vi "ReversedEngineering GetControlInfo.vi"(2 "CtlRefnum":refnum<vi>, 3 "Default Value":variant, 5 "error in":errorcluster) -> (15 "attributeInfoType":T2={"name"="", "type"=enum."UINT8", "dimension"=0, "typeName"="", "typePath"=path "", "visibility"=enum."Protected"}, 19 "error out":errorcluster)   [LabVIEW 2020]
uses:
  <resource>/Framework/Providers/Open_GDS/UML/ReversedEngineering/ReversedEngineering AttributeInfoType.ctl
  <resource>/Framework/Providers/Open_GDS/ClassProviders/Common/CommonVIs/CommonVIs_AttributeDataType.ctl
  <resource>/Framework/Providers/Open_GDS/UML/UMLEditor/UMLEditor_VisibilityType.ctl
  <vilib>/numeric/LVNumericRepresentation.ctl
  <vilib>/Utility/Data Type/Type Definitions/Data Type.ctl
  <vilib>/Utility/Data Type/NI_Data Type.lvlib
panel:
  out "representation":T1
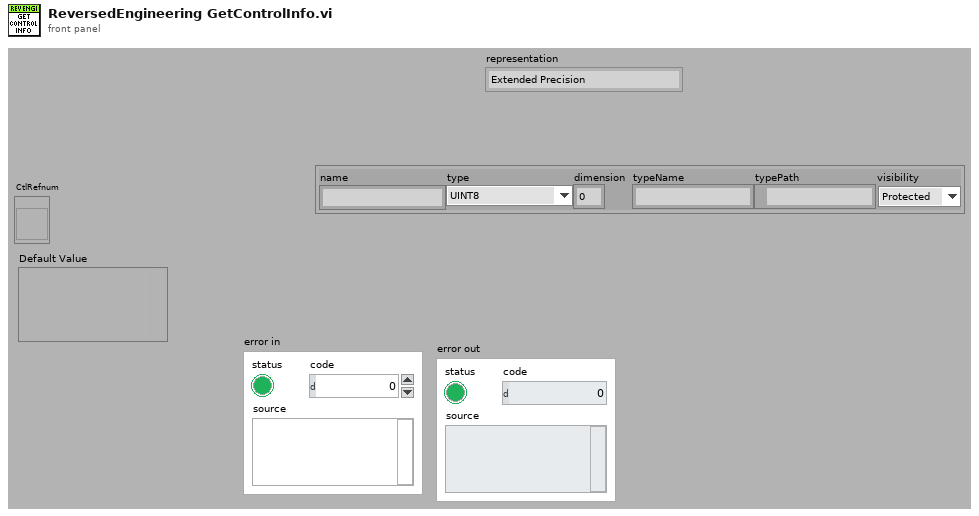
[diagram p1: front panel]
types:
  T1 = typedef "LVNumericRepresentation.ctl" = enum32{"Extended Precision", "Double Precision", "Single Precision", "Long", "Word", "Byte", "Unsigned Long", "Unsigned Word", "Unsigned Byte", "Complex Extended", "Complex Double", "Complex Single", "Quad", "Unsigned Quad", "Fixed-Point"}
  T2 = typedef "ReversedEngineering AttributeInfoType.ctl" = cluster{"name":string, "type":T3, "dimension":i32, "typeName":string, "typePath":path, "visibility":T4}
  T3 = typedef "CommonVIs_AttributeDataType.ctl" = enum16{"UINT8", "INT8", "UINT16", "INT16", "UINT32", "INT32", "UINT64", "INT64", "SGL", "DBL", "EXT", "CSG", "CDB", "CXT", "TimeStamp", "STRING", "PATH", "BOOL", "ENUM", "RefNum", "VIRefNum", "LabVIEW Class", "Cluster", "Variant", "TypeDef", "Waveform", "LabVIEW Object", "Other", "void", "Set", "Map"}
  T4 = typedef "UMLEditor_VisibilityType.ctl" = enum16{"Public", "Private", "Protected"}
  T5 = typedef "NI_Data Type.lvlib/Data Type.ctl" = enum8{"Invalid Type", "Void", "I8", "I16", "I32", "I64", "U8", "U16", "U32", "U64", "Single Float", "Double Float", "Extended Float", "Single Complex", "Double Complex", "Extended Complex", "Enum U8", "Enum U16", "Enum U32", "Enum U64", "Single Float With Unit", "Double Float With Unit", "Extended Float With Unit", "Single Complex with Unit", "Double Complex with Unit", "Extended Complex with Unit", "Boolean", "String", "Path", "Picture", "Tag", "Array", "Cluster", "Variant", "LV Variant", "Waveform", "Timestamp", "Digital Waveform", "Digital Data", "ExpressData", "Refnum", "External Data", "VI", "Poly VI", "LabVIEW Class Instance", "Fixed Point", "Set Collection", "Map Collection"}
  T6 = typedef "Member VI Info.ctl" = cluster{"qualified name":string, "path":path, "access scope":enum32{"invalid scope", "public", "private", "protected", "community"}, "is dynamic dispatch":bool}
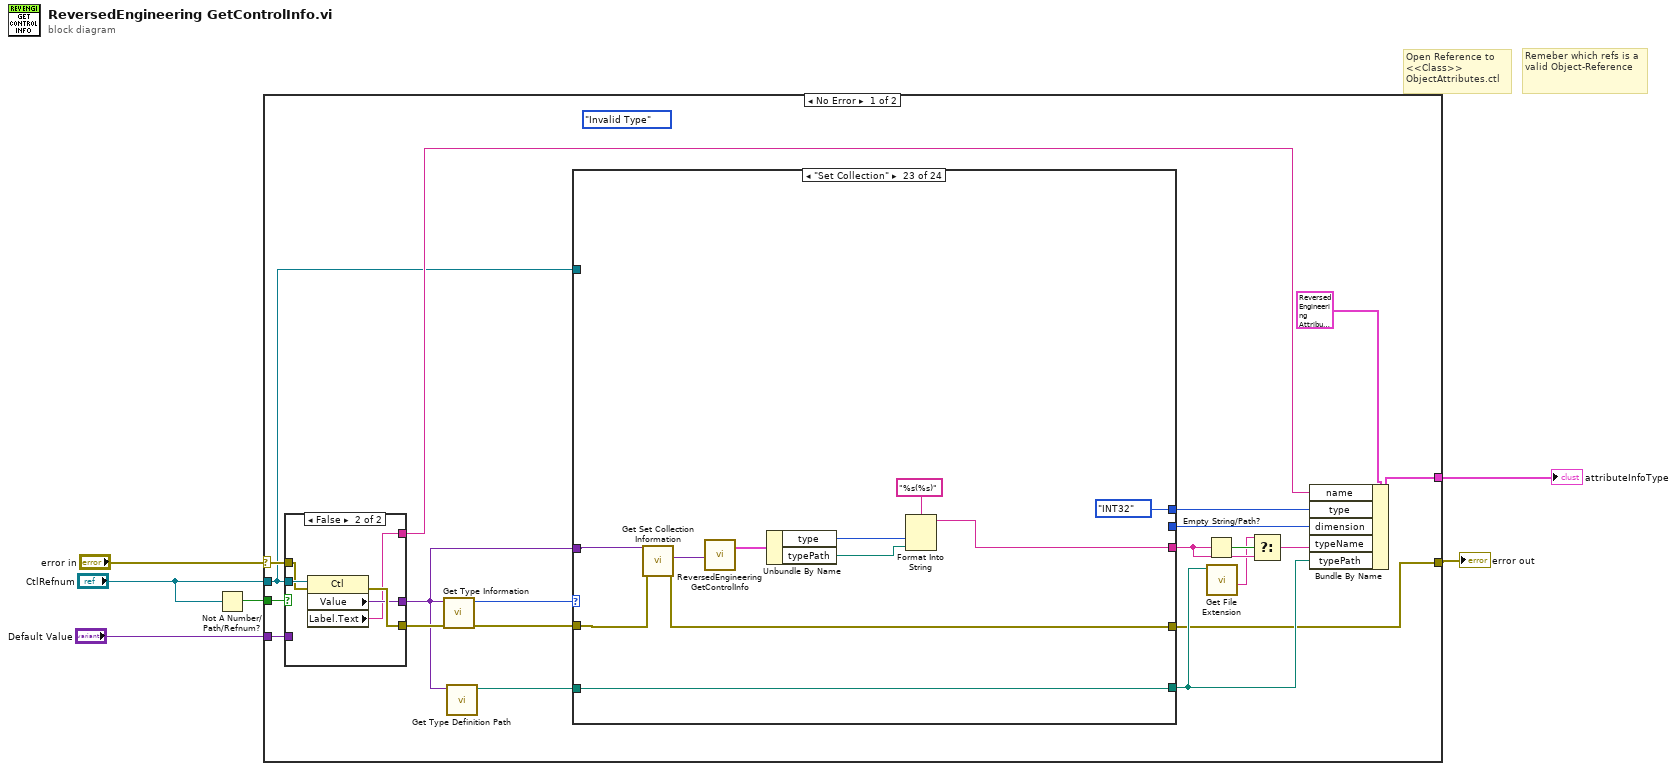
[diagram p0: block diagram]
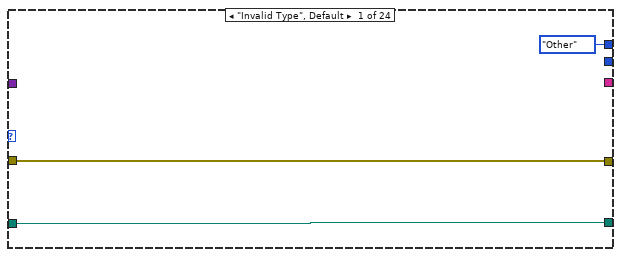
[diagram p3: hidden frame]
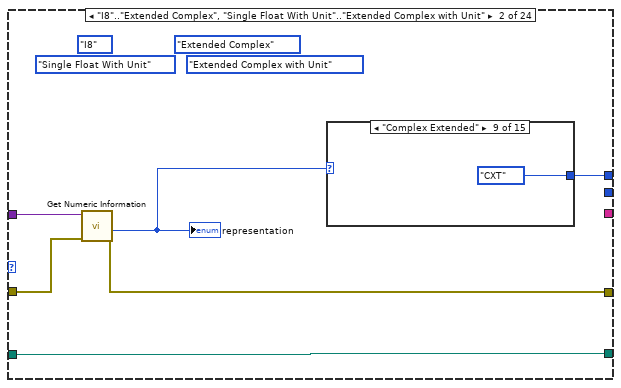
[diagram p4: hidden frame]
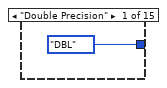
[diagram p5: hidden frame]
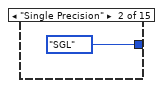
[diagram p6: hidden frame]
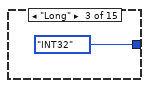
[diagram p7: hidden frame]
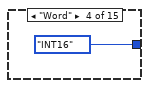
[diagram p8: hidden frame]
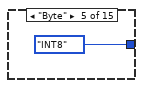
[diagram p9: hidden frame]
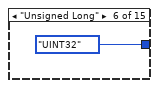
[diagram p10: hidden frame]
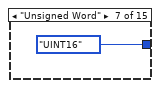
[diagram p11: hidden frame]
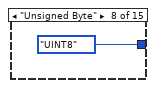
[diagram p12: hidden frame]
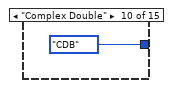
[diagram p13: hidden frame]
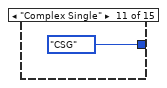
[diagram p14: hidden frame]
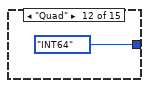
[diagram p15: hidden frame]
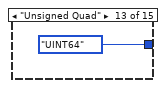
[diagram p16: hidden frame]
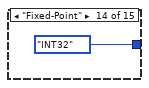
[diagram p17: hidden frame]
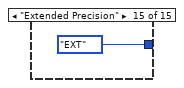
[diagram p18: hidden frame]
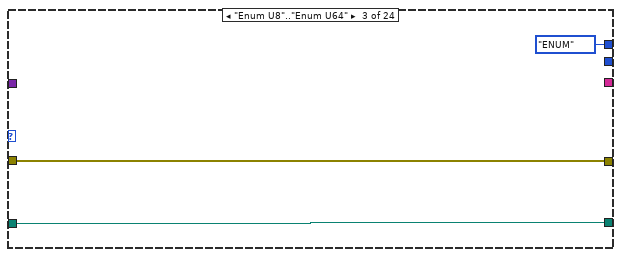
[diagram p19: hidden frame]
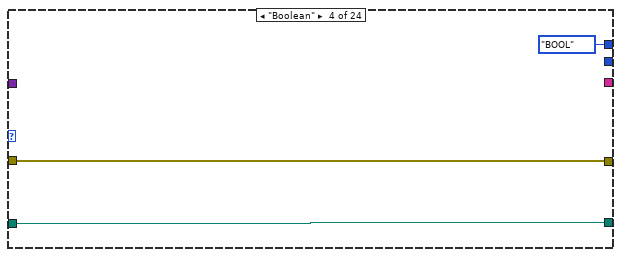
[diagram p20: hidden frame]
diagram:
  # "Remeber which refs is a valid Object-Reference"
  # "Open Reference to <<Class>> ObjectAttributes.ctl"
  n1 = Not A Number/Path/Refnum?(number/path/refnum="CtlRefnum") -> (NaN/Path/Refnum?=w2:bool)
  n2 = case shown="No Error" "error in" {
    selector: "error in" -> [w26 w175]
    tunnel: [w12 w175] -> w5
    tunnel: "CtlRefnum" -> [w7 _]
    tunnel: [w22 _] -> w4
    tunnel: w2 -> [w17 _]
    tunnel: "Default Value" -> [w16 _]
    frame No Error {
      (unwired) Data_Type."Invalid Type" ("type")
      n3 = case shown="False" w17 {
        tunnel: w7 -> [_ w33]
        tunnel: w26 -> [w27 w32]
        tunnel: [w27 w31] -> w25
        tunnel: [_ w29] -> w21
        tunnel: [w28 w30] -> w18
        tunnel: w16 -> [w28 _]
        frame True {
        }
        frame False {
          n4 = property class="Ctl"(reference=w33, error in=w32) -> (error out=w31:errorcluster, "Value"=w30:variant, "Label.Text"=w29:string)  [unwired: 1 out]
        }
      }
      n5 = call <vilib>:"Get Type Information.vi"("error in (no error)"=w25, "variant"=w18) -> ("error out"=w13:errorcluster, "type"=w24:T5)  [unwired: 5 in, 3 out]
      n6 = call <vilib>:"Get Type Definition Path.vi"("variant"=w18) -> ("type definition path"=w15:path)  [unwired: 9 in, 1 out]
      n7 = case shown="\"Set Collection\"" w24 {
        tunnel: w18 -> [_ w42 _ _ _ _ _ w84 _ _ _ _ _ _ _ _ _ _ _ _ w125 _ w157 w172]
        tunnel: w13 -> [w34 w37 w58 w61 w64 w67 w70 w75 w85 w88 w91 w94 w97 w100 w103 w106 w109 w112 w115 w118 w127 w146 w156 w171]
        tunnel: [CommonVIs_AttributeDataType."Other" ("type") w41 CommonVIs_AttributeDataType."ENUM" ("type") CommonVIs_AttributeDataType."BOOL" ("type") CommonVIs_AttributeDataType."STRING" ("type") CommonVIs_AttributeDataType."PATH" ("type") CommonVIs_AttributeDataType."STRING" ("type") w76 CommonVIs_AttributeDataType."Cluster" ("type") CommonVIs_AttributeDataType."Variant" ("type") CommonVIs_AttributeDataType."Variant" ("type") CommonVIs_AttributeDataType."Waveform" ("type") CommonVIs_AttributeDataType."TimeStamp" ("type") CommonVIs_AttributeDataType."Waveform" ("type") CommonVIs_AttributeDataType."Other" ("type") CommonVIs_AttributeDataType."Other" ("type") CommonVIs_AttributeDataType."RefNum" ("type") CommonVIs_AttributeDataType."Other" ("type") CommonVIs_AttributeDataType."VIRefNum" ("type") CommonVIs_AttributeDataType."VIRefNum" ("type") CommonVIs_AttributeDataType."LabVIEW Class" ("type") CommonVIs_AttributeDataType."INT32" ("type") CommonVIs_AttributeDataType."INT32" ("type") CommonVIs_AttributeDataType."Map" ("type")] -> w20
        tunnel: [_ _ _ _ _ _ _ w83 _ _ _ _ _ _ _ _ _ _ _ _ _ _ _ _] -> w19
        tunnel: w15 -> [w36 w39 w59 w62 w65 w68 w71 w78 w86 w89 w92 w95 w98 w101 w104 w107 w110 w113 w116 w119 _ w147 w158 w173]
        tunnel: [w36 w39 w59 w62 w65 w68 w71 w77 w86 w89 w92 w95 w98 w101 w104 w107 w110 w113 w116 w119 w121 w147 w158 w173] -> w14
        tunnel: [w34 w38 w58 w61 w64 w67 w70 w73 w85 w88 w91 w94 w97 w100 w103 w106 w109 w112 w115 w118 w123 w146 w155 w170] -> w12
        tunnel: [_ _ _ _ _ _ _ _ _ _ _ _ _ _ _ _ _ _ _ _ _ _ w149 w162] -> w10
        tunnel: w7 -> [_ _ _ _ _ _ _ _ _ _ _ _ _ _ _ _ _ _ _ _ _ _ _ _]
        frame "Invalid Type", Default {
        }
        frame "I8".."Extended Complex", "Single Float With Unit".."Extended Complex with Unit" {
          (unwired) Data_Type."Extended Complex with Unit" ("type")
          (unwired) Data_Type."Single Float With Unit" ("type")
          (unwired) Data_Type."Extended Complex" ("type")
          (unwired) Data_Type."I8" ("type")
          n8 = call <vilib>:"Get Numeric Information.vi"("error in (no error)"=w37, "variant"=w42) -> ("error out"=w38:errorcluster, "representation"=w40:T1)  [unwired: 6 in, 2 out]
          "representation" <- w40
          n9 = case shown="\"Complex Extended\"" w40 {
            tunnel: [CommonVIs_AttributeDataType."DBL" ("type") CommonVIs_AttributeDataType."SGL" ("type") CommonVIs_AttributeDataType."INT32" ("type") CommonVIs_AttributeDataType."INT16" ("type") CommonVIs_AttributeDataType."INT8" ("type") CommonVIs_AttributeDataType."UINT32" ("type") CommonVIs_AttributeDataType."UINT16" ("type") CommonVIs_AttributeDataType."UINT8" ("type") CommonVIs_AttributeDataType."CXT" ("type") CommonVIs_AttributeDataType."CDB" ("type") CommonVIs_AttributeDataType."CSG" ("type") CommonVIs_AttributeDataType."INT64" ("type") CommonVIs_AttributeDataType."UINT64" ("type") CommonVIs_AttributeDataType."INT32" ("type") CommonVIs_AttributeDataType."EXT" ("type")] -> w41
            frame "Double Precision" {
            }
            frame "Single Precision" {
            }
            frame "Long" {
            }
            frame "Word" {
            }
            frame "Byte" {
            }
            frame "Unsigned Long" {
            }
            frame "Unsigned Word" {
            }
            frame "Unsigned Byte" {
            }
            frame "Complex Extended" {
            }
            frame "Complex Double" {
            }
            frame "Complex Single" {
            }
            frame "Quad" {
            }
            frame "Unsigned Quad" {
            }
            frame "Fixed-Point" {
            }
            frame "Extended Precision" {
            }
          }
        }
        frame "Enum U8".."Enum U64" {
        }
        frame "Boolean" {
        }
        frame "String" {
        }
        frame "Path" {
        }
        frame "Picture" {
        }
        frame "Array" {
          n10 = call <vilib>:"Get Array Information.vi"("error in (no error)"=w75, "variant"=w84) -> ("error out"=w74:errorcluster, "array element data type"=w82:variant, "number of dimensions"=w83:i32)  [unwired: 6 in, 1 out]
          n11 = call <resource>:"ReversedEngineering GetControlInfo.vi"("Default Value"=w82, "error in"=w74) -> ("attributeInfoType"=w81:T2, "error out"=w73:errorcluster)  [unwired: 16 in]
          n12 = Unbundle By Name(w81) -> ("type"=w76:T3, "typePath"=w79:path)
          n13 = Empty String/Path?(string/path=w78) -> (empty?=w80:bool)
          n14 = Select(t=w79, s=w80, f=w78) -> (s? t:f=w77:path)
        }
        frame "Cluster" {
        }
        frame "Variant" {
        }
        frame "LV Variant" {
        }
        frame "Waveform" {
        }
        frame "Timestamp" {
        }
        frame "Digital Waveform" {
        }
        frame "Digital Data" {
        }
        frame "ExpressData" {
        }
        frame "Refnum" {
        }
        frame "External Data" {
        }
        frame "VI" {
        }
        frame "Poly VI" {
        }
        frame "LabVIEW Class Instance" {
          n15 = Variant To Data(error in=w127, type=refnum<class> refnum ("object"), Variant=w125) -> (data=w122:refnum<class>, error out=w124:errorcluster)
          n16 = case shown="Error .." w124 {
            selector: w124 -> [w130 w134]
            tunnel: w125 -> [_ w135]
            tunnel: [w129 w134] -> w123
            tunnel: w122 -> [w132 _]
            tunnel: [w131 w133] -> w121
            frame No Error {
              n17 = call <vilib>:"Get LV Class Path.vi"("error in (no error)"=w130, "object"=w132) -> ("error out"=w129:errorcluster, "class path"=w131:path)  [unwired: 8 in]
            }
            frame Error {
              n18 = call <vilib>:"Get LabVIEW Class Parent And Member VI Information.vi"("variant"=w135) -> ("member VI info"=w136:T6[])  [unwired: 7 in, 3 out]
              n19 = for {
                tunnel: w136 -> [w145] mode=indexing
                tunnel: [w139] -> w133
                stop <- w143 continue-if-true
                n20 = Unbundle By Name(w145) -> ("path"=w138:path)
                n21 = Strip Path(path=w138) -> (stripped path=w137:path)  [unwired: 1 out]
                n22 = List Folder(path=w137, pattern="*.lvclass") -> (path out=w141:path, filenames=w142:string[])  [unwired: 2 in, 2 out]
                n23 = Empty Array?(array=w142) -> (empty?=w143:bool)
                n24 = Index Array(array=w142) -> (element=w140:string)  [unwired: 1 in]
                n25 = Build Path(base path=w141, name or relative path=w140) -> (appended path=w139:path)
              }
            }
          }
        }
        frame "Fixed Point" {
        }
        frame "Set Collection" {
          n26 = call <vilib>:"Get Set Collection Information.vi"("error in (no error)"=w156, "variant"=w157) -> ("error out"=w155:errorcluster, "element data type"=w154:variant)  [unwired: 8 in]
          n27 = call <resource>:"ReversedEngineering GetControlInfo.vi"("Default Value"=w154) -> ("attributeInfoType"=w153:T2)  [unwired: 17 in, 1 out]
          n28 = Unbundle By Name(w153) -> ("type"=w152:T3, "typePath"=w150:path)
          n29 = Format Into String(format string="%s(%s)", w152, w150) -> (resulting string=w149:string)  [unwired: 2 in, 1 out]
        }
        frame "Map Collection" {
          n30 = call <vilib>:"Get Map Collection Information.vi"("error in (no error)"=w171, "variant"=w172) -> ("error out"=w170:errorcluster, "value data type"=w163:variant, "key data type"=w165:variant)  [unwired: 7 in]
          n31 = call <resource>:"ReversedEngineering GetControlInfo.vi"("Default Value"=w165) -> ("attributeInfoType"=w169:T2)  [unwired: 17 in, 1 out]
          n32 = call <resource>:"ReversedEngineering GetControlInfo.vi"("Default Value"=w163) -> ("attributeInfoType"=w164:T2)  [unwired: 17 in, 1 out]
          n33 = Unbundle By Name(w169) -> ("type"=w168:T3, "typePath"=w166:path)
          n34 = Unbundle By Name(w164) -> ("type"=w161:T3, "typePath"=w160:path)
          n35 = Format Into String(format string="%s(%s),%s(%s)", w168, w166, w161, w160) -> (resulting string=w162:string)  [unwired: 2 in, 1 out]
        }
      }
      n36 = Empty String/Path?(string/path=w10) -> (empty?=w11:bool)
      n37 = call <vilib>:"Get File Extension.vi"("file"=w14) -> ("filename without extension"=w9:string)  [unwired: 6 in, 4 out]
      n38 = Select(t=w9, s=w11, f=w10) -> (s? t:f=w8:string)
      n39 = Bundle By Name(cluster=T2 {"name"="", "type"=enum."UINT8", "dimension"=0, "typeName"="", "typePath"=path "", "visibility"=enum."Protected"} ("attributeInfoType"), "name"=w21, "type"=w20, "dimension"=w19, "typeName"=w8, "typePath"=w14) -> (w22:T2)
    }
    frame Error {
    }
  }
  "attributeInfoType" <- w4
  "error out" <- w5
